vi "filename.vi"() -> ()   [LabVIEW 2016]
panel:
  out "filename_global":string
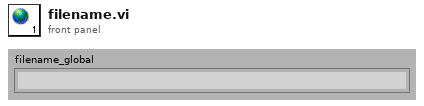
[diagram p1: front panel]
diagram:
